vi "Set DUT SIM Slot IMS Supported.vi"(7 "IMS (On)":bool=TRUE, 8 "error in (no error)":errorcluster, 9 "SIM Slot (1)":i32=1, 10 "DUT (\"DUT1\")":string="DUT1", 11 "VISA resource name":refnum<visa-resource-name>) -> (0 "error out":errorcluster, 3 "VISA resource name out":refnum<visa-resource-name>)   [LabVIEW 2015, in "Rohde&Schwarz CMXP Base.lvlib"]
doc: "Selects whether the inactive DUT supports IP multimedia subsystem (IMS) services.\n\nAttribute:\nRSCMXPBASE_ATTR_SELECT_DUT_SIM_SLOT\n\nRemote-control command:\n[CONFigure:]DUT:PROFile:SIMSlot<no>:CAPability:IMS"
uses:
  <instrlib>/Rohde&Schwarz CMXP Base/Rohde&Schwarz CMXP Base.lvlib
  <instrlib>/Rohde&Schwarz CMXP Base/Private/rsidr_core.llb/rsidr_core.lvlib
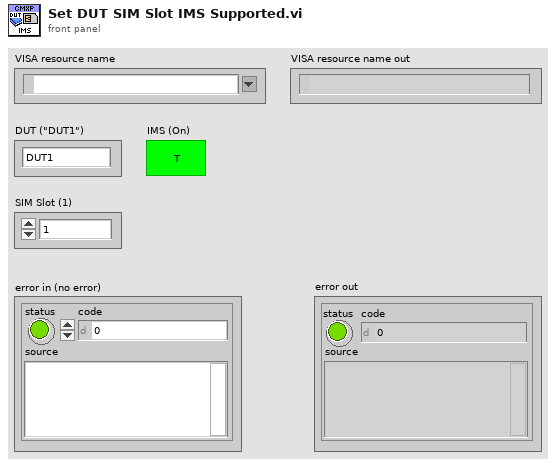
[diagram p1: front panel]
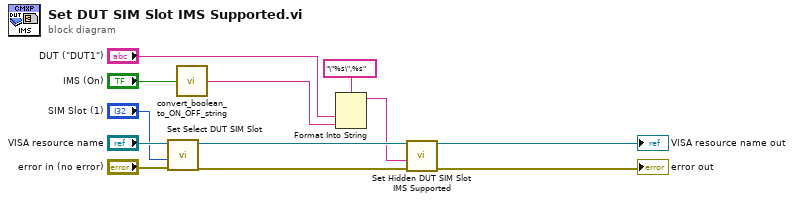
[diagram p0: block diagram]
diagram:
  n1 = call "Set Select DUT SIM Slot"("error in (no error)"="error in (no error)", "Select DUT SIM Slot (0)"="SIM Slot (1)", "instrument handle"="VISA resource name") -> ("error out"=w3:errorcluster, "instrument handle out"=w5:refnum<visa-resource-name>)  [unwired: 7 in]
  n2 = call <instrlib>:"convert_boolean_to_ON_OFF_string.vi"("boolean value in"="IMS (On)") -> ("string value out"=w4:string)  [unwired: 4 in]
  n3 = Format Into String(format string="\"%s\",%s", "DUT (\"DUT1\")", w4) -> (resulting string=w2:string)  [unwired: 2 in, 1 out]
  n4 = call "Set Hidden DUT SIM Slot IMS Supported"("error in (no error)"=w3, "Hidden DUT SIM Slot IMS Supported ()"=w2, "instrument handle"=w5) -> ("error out"=→"error out":errorcluster, "instrument handle out"=→"VISA resource name out":refnum<visa-resource-name>)  [unwired: 7 in]
